vi "Test Suite from Project.vi"(8 "error in (no error)":errorcluster, 11 "Test Case In":refnum<class "LUnit Test Suite Tests.lvclass">) -> (0 "error out":errorcluster, 3 "Test Case Out":refnum<class "LUnit Test Suite Tests.lvclass">)   [LabVIEW 2020, in "LUnit Test Suite Tests.lvclass"]
uses:
  LUnit Test Suite Tests.lvclass
  C:/Program Files (x86)/National Instruments/LabVIEW 2020/vi.lib/Astemes/LUnit/Test Case.lvclass
  Result/Type.ctl
  Light Test Case Double/Light Test Case Double.lvclass
  <vilib>/Astemes/LUnit/Test Case.lvclass/Test Case.ctl
  b74e4934-f044-4222-b3dd-fc90e6c1bd4f.vi
  <vilib>/Astemes/LUnit/Palette/Pass.vi
  <vilib>/Astemes/LUnit/Palette/Fail.vi
  <vilib>/Astemes/LUnit/Compare Variants.vi
  <vilib>/Astemes/LUnit/Describe Comparison.vi
  <vilib>/Astemes/LUnit/Set Assertion Type.vi
  <vilib>/Astemes/LUnit/Add test result.vi
  <vilib>/Astemes/LUnit/Variant to string.vi
  <vilib>/Astemes/LUnit/LUnit Record Assertion Result.vi
  <vilib>/Astemes/LUnit/LUnit Aggregate Assertion Results.vi
  <vilib>/Astemes/LUnit/Method Result/LUnit Merge Status.vi
  <vilib>/Astemes/LUnit/LUnit Concatenate result strings.vi
  Mock Result Observer/Mock Result Observer.lvclass
  C:/Git/astemes-lunit/source/Rewrite Project/Result Observer/Result Observer.lvclass
  <vilib>/Utility/Data Type/Get Type Information.vi
  LUnit Test Suite/LUnit Test Suite V2.lvclass
  Result/Result.lvlib
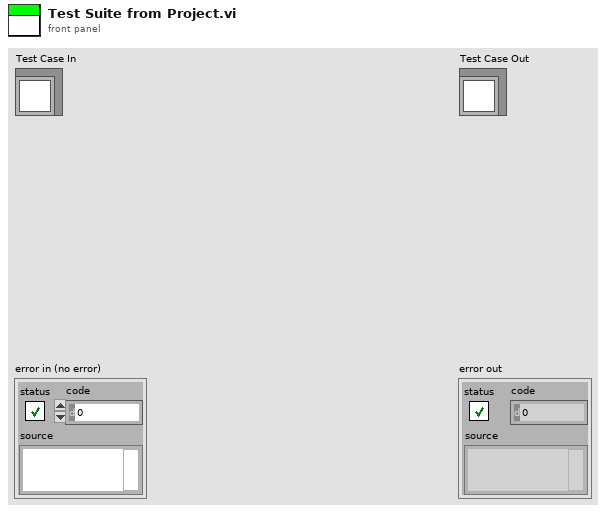
[diagram p1: front panel]
types:
  T1 = typedef "Result.lvlib/Type.ctl" = enum16{"Method", "Case", "Suite", "Pass", "Fail", "Skip", "Pass if", "Fail if", "Pass if Error", "Fail if Error", "Pass if Equal", "Fail if Equal"}
  T2 = typedef "Result.lvlib/Result.ctl" = cluster{"Case":string, "Message":string, "Description":string, "Status":T3, "Result Type":T1, "Execution Time":dbl}
  T3 = typedef "Result.lvlib/Status.ctl" = enum16{"Passed", "Failed", "Error", "Skipped", "Setup Error", "Broken", "Teardown Error"}
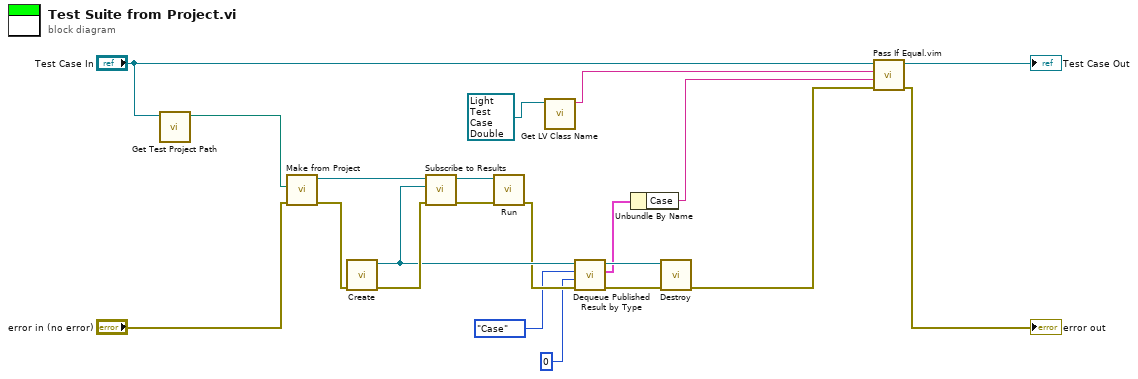
[diagram p0: block diagram]
diagram:
  n1 = call "Get Test Project Path.vi"("LUnit Test Suite Tests in"="Test Case In") -> ("appended path"=w18:path)  [unwired: 10 in]
  n2 = call "Make from Project.vi"("error in (no error)"="error in (no error)", "Project Path"=w18) -> ("error out"=w13:errorcluster, "LUnit Test Suite V2 Out"=w16:refnum<class "LUnit Test Suite V2.lvclass">)  [unwired: 8 in]
  n3 = call "Create.vi"("error in (no error)"=w13) -> ("error out"=w14:errorcluster, "Mock Result Observer out"=w12:refnum<class "Mock Result Observer.lvclass">)  [unwired: 9 in]
  n4 = call-dynamic "Subscribe to Results.vi"("error in (no error)"=w14, "Result Observer"=w12, "LUnit Test Suite V2 In"=w16) -> ("error out"=w17:errorcluster, "LUnit Test Suite V2 Out"=w15:refnum<class "LUnit Test Suite V2.lvclass">)  [unwired: 7 in]
  n5 = call-dynamic "Run.vi"("error in (no error)"=w17, "Run in"=w15) -> ("error out"=w11:errorcluster)  [unwired: 8 in, 1 out]
  n6 = call <vilib>:"Get LV Class Name.vi"("object"=refnum<class "Light Test Case Double.lvclass"> refnum ("Light Test Case Double.lvclass")) -> ("class name"=w2:string)  [unwired: 9 in, 1 out]
  n7 = call "Dequeue Published Result by Type.vi"("error in (no error)"=w11, "timeout in ms"=0, "Result Type"=Type."Case", "Mock Result Observer In"=w12) -> ("error out"=w7:errorcluster, "Result"=w5:T2, "Mock Result Observer Out"=w10:refnum<class "Mock Result Observer.lvclass">)  [unwired: 4 in, 1 out]
  n8 = Unbundle By Name(w5) -> ("Case"=w4:string)
  n9 = call "Destroy.vi"("error in (no error)"=w7, "Mock Result Observer in"=w10) -> ("error out"=w8:errorcluster)  [unwired: 9 in]
  n10 = call "Pass If Equal.vim"("error in (no error)"=w8, "Actual"=w4, "Expected"=w2, "LUnit Test Case In"="Test Case In") -> ("error out"=→"error out":errorcluster, "LUnit Test Case Out"=→"Test Case Out":refnum<class "LUnit Test Suite Tests.lvclass">)  [unwired: 6 in]
